vi "Stack Temp HMI Screen Dev.vi"() -> ()   [LabVIEW 2019]
panel:
  out "Button":bool
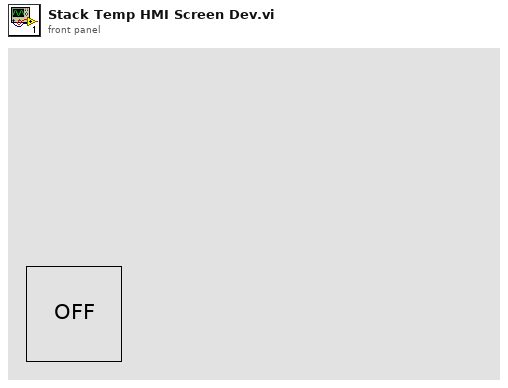
[diagram p1: front panel]
types:
  T1 = typedef "imagedata.ctl" = cluster{"image type":i32, "image depth":i32, "image":u8[], "mask":u8[], "colors":u32[], "Rectangle":cluster{"left":i16, "top":i16, "right":i16, "bottom":i16}}
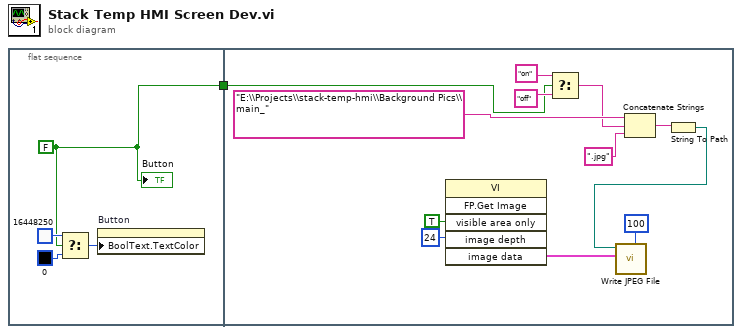
[diagram p0: block diagram]
diagram:
  n1 = flat-sequence {
    tunnel: [w2] -> w1
    tunnel: w1 -> [w7]
    frame #0 {
      w2 = FALSE ("s")
      n2 = Select(t=u32 16448250 ("Boolean Text.Text Colors:Text Color"), s=w2, f=u32 0 ("Boolean Text.Text Colors:Text Color")) -> (s? t:f=w3:u32)
      n3 = property on="Button" class="Bool"("BoolText.TextColor"=w3) -> ()  [unwired: 2 in, 2 out]
      "Button" <- w2
    }
    frame #1 {
      n4 = invoke class="VI" method="FP.Get Image"("visible area only"=TRUE ("Visible Area Only"), "image depth"=24 ("Image Depth")) -> ("image data"=w16:T1)  [unwired: 4 in, 5 out]
      n5 = Select(t="on" ("string"), s=w7, f="off" ("string")) -> (s? t:f=w6:string)
      n6 = Concatenate Strings("E:\\Projects\\stack-temp-hmi\\Background Pics\\main_", w6, ".jpg" ("string")) -> (w11:string)
      n7 = String To Path(string=w11) -> (path=w13:path)
      n8 = call <vilib>:"Write JPEG File.vi"("quality (80)"=100, "image data"=w16, "path to JPEG file"=w13) -> ()  [unwired: 7 in, 2 out]
    }
  }
